vi "Basic Amplitude Measurements.vi"() -> ()   [LabVIEW 2011]
doc: "This example shows how to take some amplitude measurements on a simulated signal. The measurements are Mean (DC) and RMS.\n\nThis example uses the following Express VIs: Simulate Signal and Amplitude and Measurements"
uses:
  Instance           1 36Saved   Basic Amplitude Measurements .vi
  Instance           2 36Saved   Basic Amplitude Measurements .vi
  Instance           3 36Saved   Basic Amplitude Measurements .vi
panel:
  in  "Frequency":dbl(slide)=100.49261083743842 scale=0.0..100.0
  out "RMS":dbl format="%0.2f"
  out "Mean":dbl format="%0.2f"
  in  "Amplitude":dbl(slide)=100.49261083743842 scale=0.0..10.0
  out "Input":dynamicdata(graph)=[{"t0"=timestamp(21.300000190734863 s since 1904-01-01), "dt"=0.001, "Y"=[-1.045426032151304, -2.5037197611687847, -2.99654825251707, -2.3338707580624307, -0.7712238975993304, 1.0888164152541084, 2.5289956815818373, 2.9939630034054576, 2.304421243387486, 0.7262662136486071, -1.1319460307379796, -2.5536659166167683, -2.990660710912945, -2.2744198281053865, -0.6811345915494608, 1.1748045492149866, 2.5777245578409334, 2.9866421659267184, 2.2438736974472886, 0.6358398401632068, -1.2173817062239638, -2.6011658432962133, -2.981908330873862, -2.2127901671017156, -0.5903928074200355, 1.2596673046888083, 2.6239841588789767, 2.976460339490859, 2.1811766814624987, 0.5448043777209927, -1.3016512173606245, -2.6461740396846314, -2.9702994965520713, -2.149040811845846, -0.49908546933116904, 1.343323389243197, 2.6677301713164625, 2.9634272775572437, 2.116390254677054, 0.4532470317648392, -1.3846738400011034, -2.688647391158405, -2.9558453283781305, -2.0832328296472395, -0.4073000431630859, 1.4256926663499743, 2.708920689611468, 2.9475554648643163, 2.0495764778405503, 0.36125550766457465, -1.4663700444282954, -2.728545211293523, -2.9385596724083207, -2.015429259832296, -0.31512445277009044, 1.5066962321501958, 2.74751625620215, 2.928860105470117, 1.980799353758502, 0.2689179267015383, -1.5466615715386023, -2.7658292808402525, -2.91845908706113, -1.9456950533572277, -0.22264699575586266, 1.5862564910383523, 2.7834798993042416, 2.9073591081878947, 1.9101247659822758, 0.17632274165475645, -1.6254715078085045, -2.800463884334419, -2.895562827255464, -1.8740970105896557, -0.1299562588906167, 1.6642972299934566, 2.8167771683274005, 2.8830730694307336, 1.8376204156973226, 0.08355865206945358, -1.7027243589722605, -2.8324158443102894, -2.869892825965822, -1.8007037173186797, -0.03714103325137693, 1.7407436915856087, 2.8473761668763835, 2.8560252534816772, 1.763355756870333, -0.009285480710701972, -1.7783461223399577, -2.8616545530821855, -2.841473673212078, -1.725585479054605, 0.05570977083351682, 1.8155226455882614, 2.875247583305507, 2.8262415702082104, 1.68740192971731, -0.10212071866640285], "attributes"=variant("NI_ChannelName"=variant(string "Sine"), "NI_ExpIsRelativeTime"=variant(bool TRUE), "NI_ExpStartTimeStamp"=variant(dbl 3101836871.808), "NI_ExpTimeStamp"=variant(dbl 3101836893.1080003), "NI_ExpXDimension"=variant(string "t"))}]
  in  "stop":bool
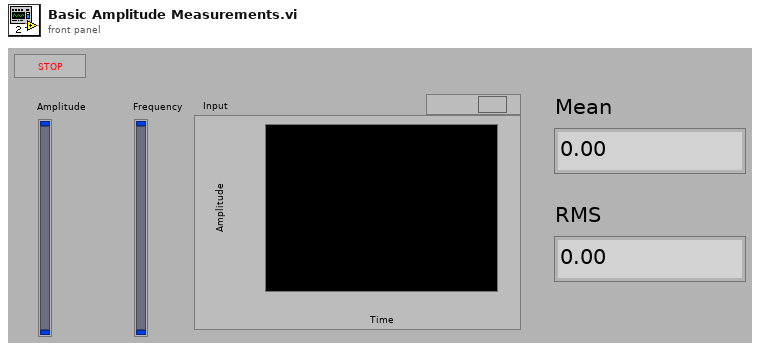
[diagram p1: front panel]
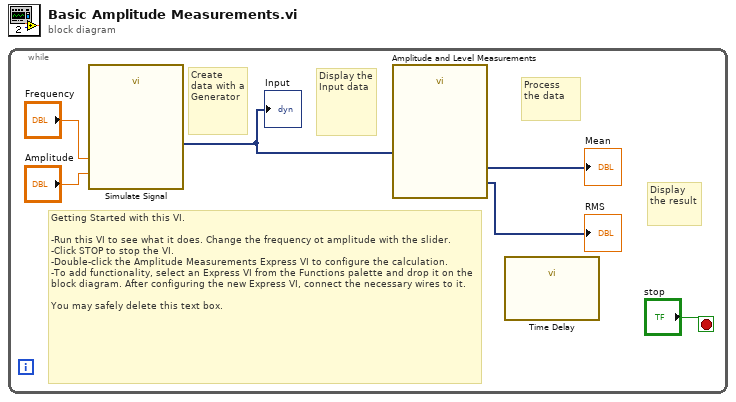
[diagram p0: block diagram]
diagram:
  n1 = while {
    stop <- "stop" stop-if-true
    # "Getting Started with this VI.\n\n-Run this VI to see what it does. Change the frequency ot amplitude with the slider.\n-Click STOP to stop the VI.\n-Double-click the Amplitude Measurements Express VI to configure the calculation.\n-To add functionality, select an Express VI from the Functions palette and drop it on the block diagram. After configuring the new Express VI, connect the necessary wires to it.\n\nYou may safely delete this text box."
    # "Display the Input data"
    # "Create data with a Generator"
    # "Process the data"
    # "Display the result"
    n2 = call "Simulate Signal"("Frequency"="Frequency", "Amplitude"="Amplitude") -> ("Sine"=w3:dynamicdata)  [unwired: 4 in, 9 out]
    "Input" <- w3
    n3 = call "Amplitude and Level Measurements"("Signals"=w3) -> ("Mean (DC)"=→"Mean":dynamicdata, "RMS"=→"RMS":dynamicdata)  [unwired: 2 in, 11 out]
    n4 = call "Time Delay"() -> ()  [unwired: 2 in, 10 out]
  }
